vi "Calculate Voltage.vi"() -> ()   [LabVIEW 2018]
uses:
  <vilib>/LabVIEW Interface for Arduino/Type Defs/Connection Type.ctl
  <vilib>/LabVIEW Interface for Arduino/LabVIEW Interface for Arduino.lvlib
panel:
  out "숫자형":dbl
  in  "정지":bool
  out "웨이브폼 차트":dbl(graph)
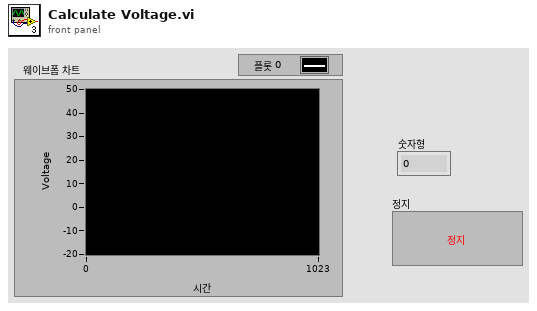
[diagram p1: front panel]
types:
  T1 = typedef "LabVIEW Interface for Arduino.lvlib/Connection Type.ctl" = enum8{"USB / Serial", "XBEE", "BlueSmirf (Bluetooth)"}
  T2 = typedef "LabVIEW Interface for Arduino.lvlib/Arduino Resource.ctl" = cluster{"VISA resource":refnum<visa-resource-name>, "Board Type":T3, "Connection Type":enum8{"USB / Serial"}, "Bytes Per Packet (15)":u8}
  T3 = typedef "LabVIEW Interface for Arduino.lvlib/Board Type.ctl" = enum16{"Uno", "Dimuelanove w/Atmega 328", "Mega 2560"}
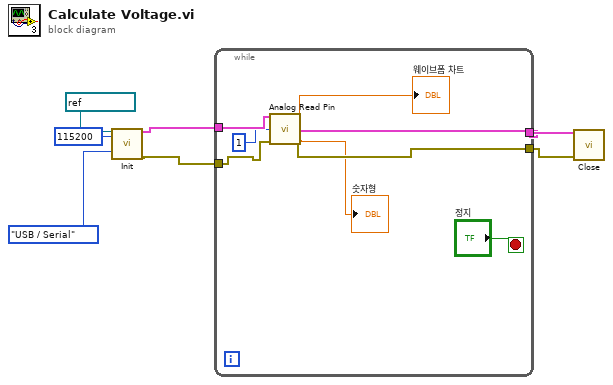
[diagram p0: block diagram]
diagram:
  n1 = call <vilib>:"Init.vi"("VISA resource"=refnum<visa-resource-name> "COM24", "Baud Rate (115200)"=u32 115200, "Connection Type (USB/Serial)"=Connection_Type."USB / Serial") -> ("Arduino Resource"=w2:T2, "error out"=w1:errorcluster)  [unwired: 15 in]
  n2 = while {
    tunnel: [w11] -> w5
    tunnel: [w13] -> w3
    tunnel: w2 -> [w10]
    tunnel: w1 -> [w9]
    stop <- "정지" stop-if-true
    n3 = call <vilib>:"Analog Read Pin.vi"("Arduino Resource"=w10, "Analog Input Pin (0)"=u8 1, "error in"=w9) -> ("Arduino Resource"=w11:T2, "Voltage"=→"웨이브폼 차트" →"숫자형":dbl, "error out"=w13:errorcluster)  [unwired: 10 in]
  }
  n4 = call <vilib>:"Close.vi"("Arduino Resource"=w5, "error in"=w3) -> ()  [unwired: 13 in, 1 out]
